vi "basicEx.vi"() -> ()   [LabVIEW 2017]
uses:
  <instrlib>/BK Precision 85XX Series/BK Precision 85XX Series.lvlib
panel:
  in  "Enable Input Terminals (F: Off)":bool
  in  "VISA resource name":refnum<visa-resource-name>="COM4"
  out "error out":errorcluster
  out "Serial Number":string
  out "Product Model":string
  out "Firmware Version":string
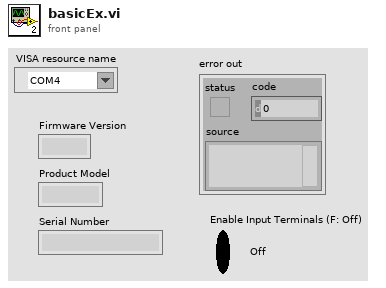
[diagram p1: front panel]
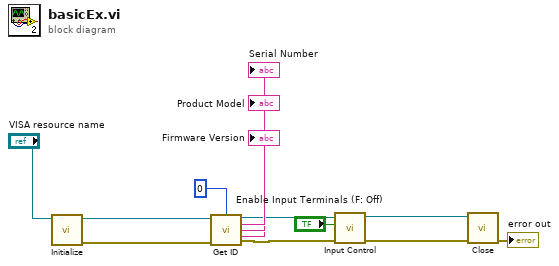
[diagram p0: block diagram]
diagram:
  n1 = call <instrlib>:"Initialize.vi"("VISA resource name"="VISA resource name") -> ("error out"=w8:errorcluster, "VISA resource name out"=w9:refnum<visa-resource-name>)  [unwired: 9 in]
  n2 = call <instrlib>:"Get ID.vi"("VISA resource name"=w9, "Communication Address (0)"=u8 0, "error in (no error)"=w8) -> ("VISA resource name out"=w2:refnum<visa-resource-name>, "Firmware Version"=→"Firmware Version":string, "Product Model"=→"Product Model":string, "Serial Number"=→"Serial Number":string, "error out"=w3:errorcluster)  [unwired: 8 in]
  n3 = call <instrlib>:"Input Control.vi"("error in (no error)"=w3, "Enable Input Terminals (F: Off)"="Enable Input Terminals (F: Off)", "VISA resource name"=w2) -> ("error out"=w4:errorcluster, "VISA resource name out"=w5:refnum<visa-resource-name>)  [unwired: 7 in]
  n4 = call <instrlib>:"Close.vi"("error in (no error)"=w4, "VISA resource name"=w5) -> ("error out"=→"error out":errorcluster)  [unwired: 9 in]
